vi "Set Output Amplitude.vi"(6 "Output channel":i32, 8 "error in (no error)":errorcluster, 10 "Output amplitude":dbl=1.0 min=-1.0 max=1.0 format="%#_8pV", 11 "RP Instrument in":refnum<class "RP Instrument.lvclass">) -> (0 "error out":errorcluster, 2 "Actual output amplitude":dbl=1.0 min=-1.0 max=1.0 format="%#_8pV", 3 "RP Instrument out":refnum<class "RP Instrument.lvclass">)   [LabVIEW 2024, in "RP Instrument.lvclass"]
uses:
  RP Instrument.lvclass
  RP Command.ctl
  SoftwareLockin/Sqrt2.ctl
  RP Instrument.lvclass/RP Instrument.ctl
  RP Communicator/RP Communicator.lvclass
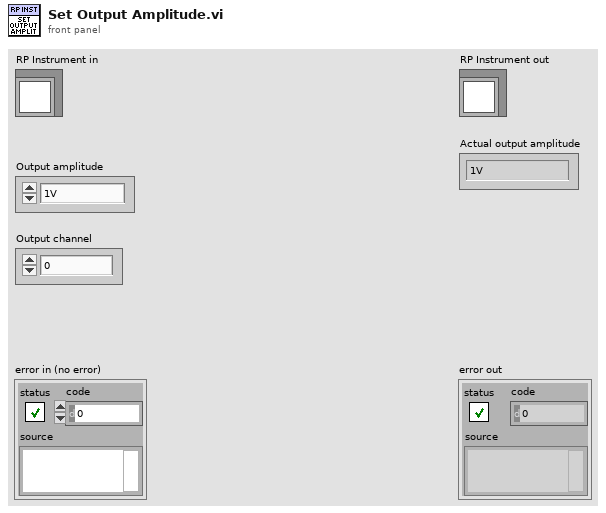
[diagram p1: front panel]
types:
  T1 = typedef "RP Command.ctl" = enum16{"Reset", "Read IDN", "Stop server", "Get status", "Get temperature", "Connect client", "Arm", "Software trigger", "Get whole buffer", "Get chunk", "System call", "Get config", "Set config", "Recieve data", "Recieve Calibartion", "Transmit data"}
  T2 = typedef "Sqrt2.ctl" = dbl
  T3 = typedef "RP Calibration.ctl" = cluster{"dataStructureId":u8, "wpCheck":u8, "fast_adc_count_1_1":u16, "padding":u32, "fast_adc_1_1":T4, "fast_adc_filter_1_1":T6, "fast_adc_count_1_20":u64, "fast_adc_1_20":T4, "fast_adc_filter_1_20":T6, "fast_adc_count_1_1_ac":u64, "fast_adc_1_1_ac":T4, "fast_adc_count_1_20_ac":u64, "fast_adc_1_20_ac":T4, "fast_dac_count_x1":u64, "fast_dac_x1":T8, "fast_dac_count_x5":u64, "fast_dac_x5":T8}
  T4 = typedef "RP Calibration 4ch.ctl" = cluster{"ch_0":T5, "ch_1":T5, "ch_2":T5, "ch_3":T5}
  T5 = typedef "RP Channel Calibration.ctl" = cluster{"baseScale":sgl, "calibValue":u32, "offset":i32, "padding 2":i32, "gainCalc":dbl}
  T6 = typedef "RP Filter 4ch.ctl" = cluster{"ch_0":T7, "ch_1":T7, "ch_2":T7, "ch_3":T7}
  T7 = typedef "RP Channel Filter.ctl" = cluster{"aa":u32, "bb":u32, "pp":u32, "kk":u32}
  T8 = typedef "RP Calibration 2ch.ctl" = cluster{"ch_0":T5, "ch_1":T5}
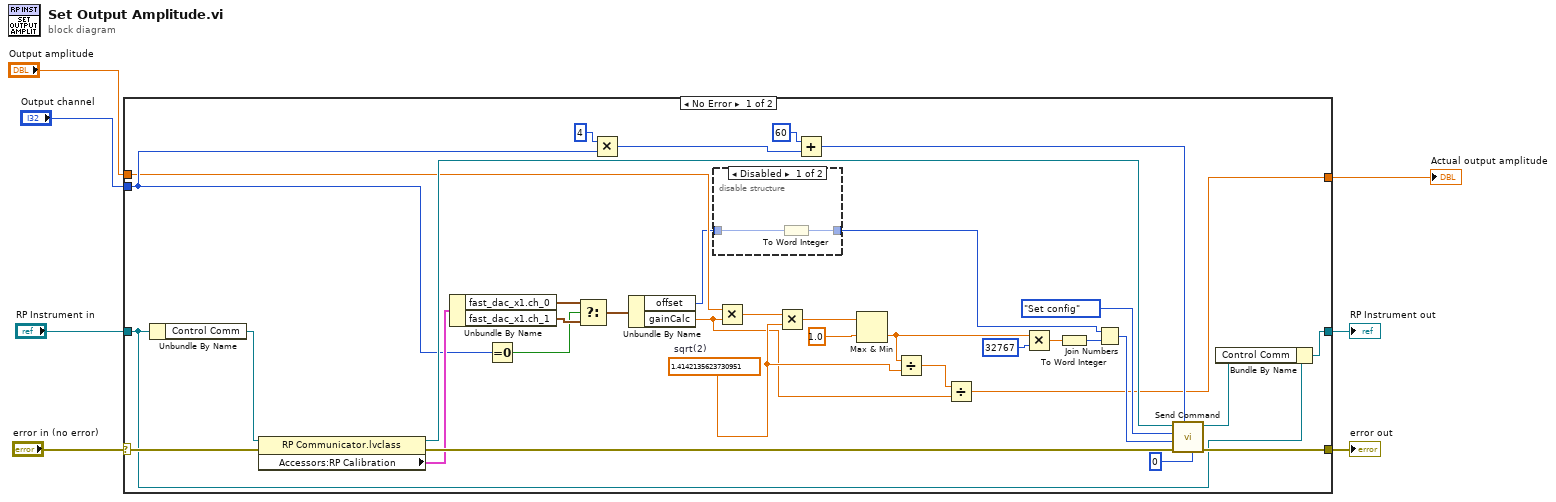
[diagram p0: block diagram]
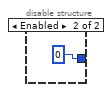
[diagram p2: hidden frame]
diagram:
  n1 = case shown="No Error" "error in (no error)" {
    selector: "error in (no error)" -> [w42 w48]
    tunnel: [w41 w48] -> w6
    tunnel: [w38 w47] -> w4
    tunnel: "RP Instrument in" -> [w40 w47]
    tunnel: "Output amplitude" -> [w20 w46]
    tunnel: "Output channel" -> [w23 _]
    tunnel: [w8 w46] -> w1
    frame No Error {
      w11 = T2 1.4142135623730951  # sqrt(2)
      n2 = Unbundle By Name(w40) -> ("Control Comm"=w28:refnum<class "RP Communicator.lvclass">)
      n3 = property class="RP Communicator.lvclass"(reference=w28, error in=w42) -> (reference out=w27:refnum<class "RP Communicator.lvclass">, error out=w29:errorcluster, "Accessors:RP Calibration"=w26:T3)
      n4 = Unbundle By Name(w26) -> ("fast_dac_x1.ch_0"=w25:T5, "fast_dac_x1.ch_1"=w24:T5)
      n5 = Equal To 0?(x=w23) -> (x = 0?=w22:bool)
      n6 = Select(t=w25, s=w22, f=w24) -> (s? t:f=w21:T5)
      n7 = Multiply(x=4, y=w23) -> (x*y=w31:i32)
      n8 = Unbundle By Name(w21) -> ("offset"=w18:i32, "gainCalc"=w9:dbl)
      n9 = disable-structure shown="Disabled" {
        disable-tunnel: w18 -> [w44 _]
        disable-tunnel: [w43 i16 0] -> w17
        frame Disabled {
          n10 = To Word Integer(number=w44) -> (16bit integer=w43:i16)
        }
        frame Enabled {
        }
      }
      n11 = Multiply(x=w20, y=w9) -> (x*y=w19:dbl)
      n12 = Multiply(x=w19, y=w11) -> (x*y=w14:T2)
      n13 = Add(x=60, y=w31) -> (x+y=w30:i32)
      n14 = Max & Min(x=w14, y=1.0) -> (min(x,y)=w12:T2)  [unwired: 1 out]
      n15 = Divide(x=w12, y=w11) -> (x/y=w10:T2)
      n16 = Divide(x=w10, y=w9) -> (x/y=w8:T2)
      n17 = Multiply(x=w12, y=i16 32767) -> (x*y=w16:T2)
      n18 = To Word Integer(number=w16) -> (16bit integer=w35:i16)
      n19 = Join Numbers(hi=w17, lo=w35) -> ((hi.lo)=w36:u32)
      n20 = call-dynamic "Send Command.vi"("bytes to read"=0, "Config offset"=w30, "error in (no error)"=w29, "Command payload"=w36, "Command number"=RP_Command."Set config", "RP Communicator in"=w27) -> ("error out"=w41:errorcluster, "RP Communicator out"=w39:refnum<class "RP Communicator.lvclass">)  [unwired: 3 in, 1 out]
      n21 = Bundle By Name(cluster=w40, "Control Comm"=w39) -> (w38:refnum<class "RP Instrument.lvclass">)
    }
    frame Error {
    }
  }
  "error out" <- w6
  "RP Instrument out" <- w4
  "Actual output amplitude" <- w1
